vi "11 CommonSerialCheck.vi"(8 "error in (no error)":errorcluster caption="错误输入（无错误）", 10 "串口输入":refnum<visa-resource-name>, 11 "SerialClass 输入":refnum<class "SerialClass.lvclass">) -> (0 "error out":errorcluster caption="错误输出", 2 "同一串口？":bool, 3 "SerialClass 输出":refnum<class "SerialClass.lvclass">)   [LabVIEW 2019, in "SerialClass.lvclass"]
uses:
  SerialClass.lvclass
  SerialClass.lvclass/SerialClass.ctl
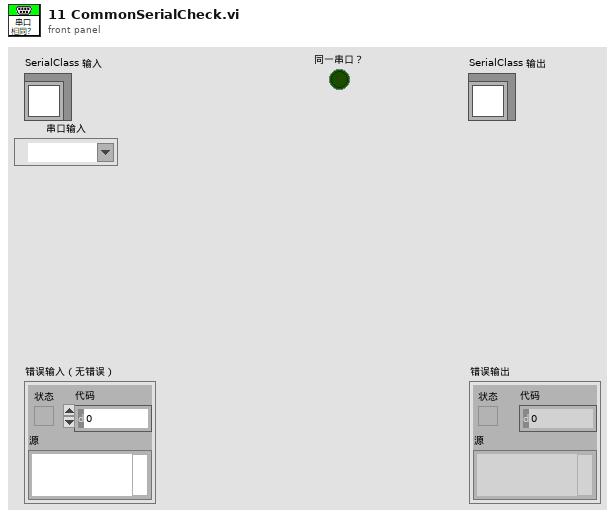
[diagram p1: front panel]
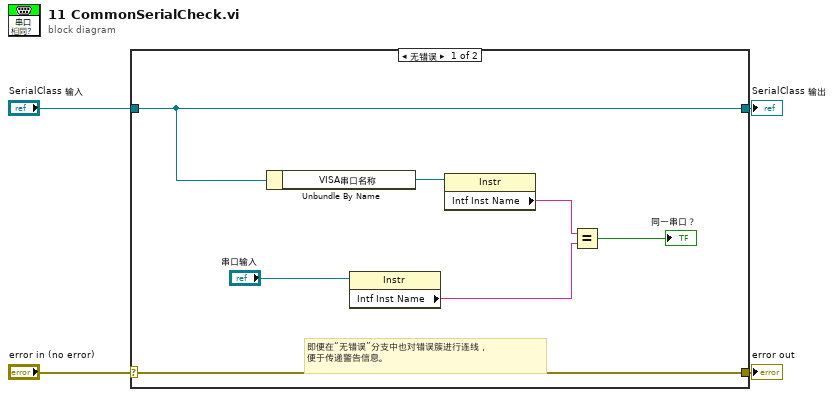
[diagram p0: block diagram]
diagram:
  n1 = case shown="无错误" "error in (no error)" {
    selector: "error in (no error)" -> [w11 w13]
    tunnel: [w11 w13] -> w3
    tunnel: [w10 w12] -> w1
    tunnel: "SerialClass 输入" -> [w10 w12]
    frame No Error {
      # "即便在“无错误”分支中也对错误簇进行连线，\n便于传递警告信息。"
      n2 = Unbundle By Name(w10) -> ("VISA串口名称"=w8:refnum<visa-resource-name>)
      n3 = property class="Instr"(reference="串口输入") -> ("Intf Inst Name"=w6:string)  [unwired: 1 in, 2 out]
      n4 = property class="Instr"(reference=w8) -> ("Intf Inst Name"=w7:string)  [unwired: 1 in, 2 out]
      n5 = Equal?(x=w7, y=w6) -> (x = y?=→"同一串口？":bool)
    }
    frame Error {
    }
  }
  "error out" <- w3
  "SerialClass 输出" <- w1
